vi "Drive Encoder Input.vi"   [LabVIEW 2009]
uses:
  Motor Encoder Global.vi
  <vilib>/eio/EIONode/EIONode.xnode
  <vilib>/rvi/eio/nirviEIOImplementation/nirviEIOImplementation.xnode
  <vilib>/rvi/eio/common/nirviEmuTemplateMethod_noerrors.vi
  <vilib>/rvi/eio/common/nirviEmuClasses.ctl
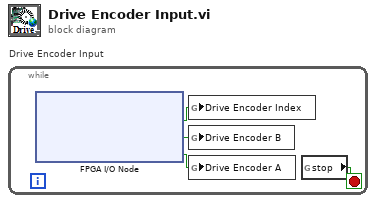
[diagram p0: block diagram]
diagram:
  n1 = while "Drive Encoder Input" {
    stop <- w1 stop-if-true
    n2 = xnode "FPGA I/O Node"() -> ("Drive Encoder Index"=w4:bool, "Drive Encoder B"=w3:bool, "Drive Encoder A"=w2:bool)  [unwired: 3 in, 3 out]
    n3 = global write "Motor Encoder Global.vi" "Drive Encoder Index"(w4) -> ()
    n4 = global write "Motor Encoder Global.vi" "Drive Encoder B"(w3) -> ()
    n5 = global write "Motor Encoder Global.vi" "Drive Encoder A"(w2) -> ()
    n6 = global read "Motor Encoder Global.vi" "stop"() -> (w1:bool)
  }
